vi "Write Data.vi"(8 "error in (no error)":errorcluster, 10 "Base Data Lib:Data":refnum<class "Data.lvclass">, 11 "Exe Write in":refnum<class "Exe Write.lvclass">) -> (0 "error out":errorcluster, 3 "Exe Write out":refnum<class "Exe Write.lvclass">)   [LabVIEW 2016, in "File Library.lvlib" / "Exe Write.lvclass"]
uses:
  Exe Write.lvclass
  <vilib>/MSR Consulting, LLC/General Reuse/Data/Data.lvclass
  Exe Write.lvclass/Exe Write.ctl
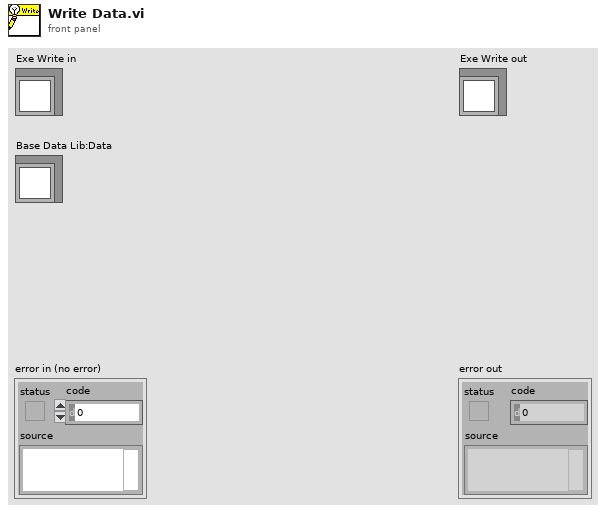
[diagram p1: front panel]
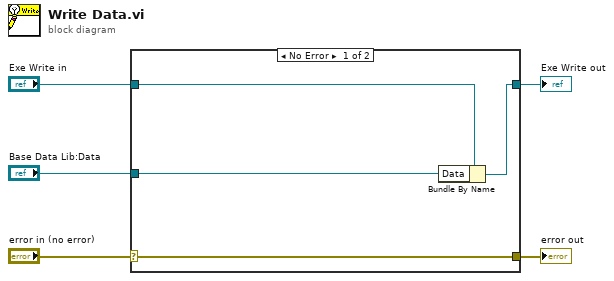
[diagram p0: block diagram]
diagram:
  n1 = case shown="No Error" "error in (no error)" {
    selector: "error in (no error)" -> [w9 w10]
    tunnel: [w9 w10] -> w4
    tunnel: [w7 w11] -> w2
    tunnel: "Exe Write in" -> [w8 w11]
    tunnel: "Base Data Lib:Data" -> [w6 _]
    frame No Error {
      n2 = Bundle By Name(cluster=w8, "Data"=w6) -> (w7:refnum<class "Exe Write.lvclass">)
    }
    frame Error {
    }
  }
  "error out" <- w4
  "Exe Write out" <- w2
